vi "Hamamatsu_serial.vi"(8 "error in":errorcluster, 9 "IMAQ Session In":refnum<k11>, 10 "Expected Response":string, 11 "Command to send":string) -> (0 "error out":errorcluster, 1 "IMAQ Session Out":refnum<k11>, 3 "Response from Camera":string)   [LabVIEW 2013]
uses:
  Experiment/Globals.vi
  Experiment/Experiment.lvclass
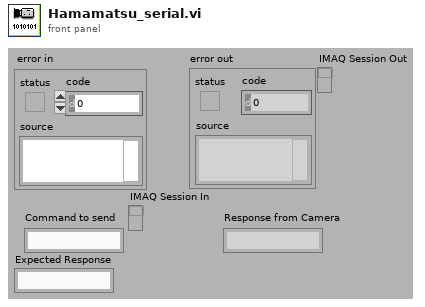
[diagram p1: front panel]
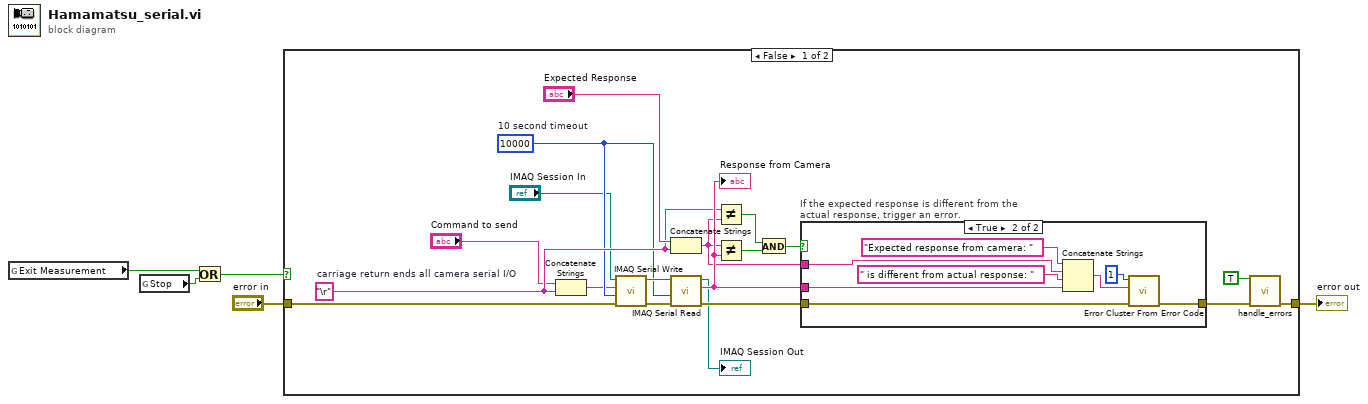
[diagram p0: block diagram]
diagram:
  n1 = global read "Globals.vi" "Exit Measurement"() -> (w2:bool)
  n2 = global read "Globals.vi" "Stop"() -> (w3:bool)
  n3 = Or(x=w2, y=w3) -> (x .or. y?=w1:bool)
  n4 = case shown="False" w1 {
    tunnel: "error in" -> [w11 w34]
    tunnel: [w7 w34] -> w4
    frame False {
      w18 = "\r"  # carriage return ends all camera serial I/O
      w14 = u32 10000  # 10 second timeout
      n5 = Concatenate Strings("Command to send", w18) -> (w13:string)
      n6 = call <vilib>:"IMAQ Serial Write.vi"("error in (no error)"=w11, "Timeout"=w14, "String to write"=w13, "IMAQ Session In"="IMAQ Session In") -> ("error out"=w17:errorcluster, "IMAQ Session Out"=w16:refnum<k11>)  [unwired: 4 in]
      n7 = Concatenate Strings("Expected Response", w18) -> (w19:string)
      n8 = call <vilib>:"IMAQ Serial Read.vi"("error in (no error)"=w17, "Timeout"=w14, "IMAQ Session In"=w16) -> ("error out"=w15:errorcluster, "String Read"=w21:string, "IMAQ Session Out"=→"IMAQ Session Out":refnum<k11>)  [unwired: 3 in, 1 out]
      "Response from Camera" <- w21
      n9 = Not Equal?(x=w18, y=w19) -> (x != y?=w23:bool)
      n10 = Not Equal?(x=w19, y=w21) -> (x != y?=w24:bool)
      n11 = And(x=w23, y=w24) -> (x .and. y?=w22:bool)
      n12 = case "If the expected response is different from the actual response, trigger an error." shown="True" w22 {
        tunnel: w15 -> [w25 w33]
        tunnel: [w25 w32] -> w8
        tunnel: w19 -> [_ w30]
        tunnel: w21 -> [_ w28]
        frame False {
        }
        frame True {
          n13 = Concatenate Strings("Expected response from camera: " ("string"), w30, " is different from actual response: " ("string"), w28) -> (w27:string)
          n14 = call <vilib>:"Error Cluster From Error Code.vi"("error in (no error)"=w33, "error message (\"\")"=w27, "error code (0)"=1) -> ("error out"=w32:errorcluster)  [unwired: 6 in]
        }
      }
      n15 = call "handle_errors.vi"("Exit Operation"=TRUE ("Exit Measurement"), "error in (no error)"=w8) -> ("error out"=w7:errorcluster)  [unwired: 13 in]
    }
    frame True {
    }
  }
  "error out" <- w4
